vi "InAs TED Characterise - VoltageInput.vi"() -> ()   [LabVIEW 2024]
uses:
  <vilib>/Analysis/1siggen.llb/Ramp Pattern by Delta.vi
  <instrlib>/Keithley DMM6500 DAQ6500 Series/Public/Data/Read (Single Point).vi
  <vilib>/Analysis/NI_AALBase.lvlib
  <instrlib>/Keithley DMM6500 DAQ6500 Series/Keithley DMM6500 DAQ6500 Series.lvlib
panel:
  in  "DMM Visa":refnum<visa-resource-name>="DMM6500"
  in  "TEC Controller":refnum<visa-resource-name>="TED4015"
  in  "Average Filter Type":i32(ring) items=["Repeat", "Moving"]
  in  "Avg Count":u32=10
  out "InAs Detector Response":cluster{"Ramp Pattern":dbl[], dbl[]}(graph)
  in  "Tdelta":dbl=1.0 format="%#_13g"
  in  "TFinish":dbl
  in  "TStart":dbl=-65.0
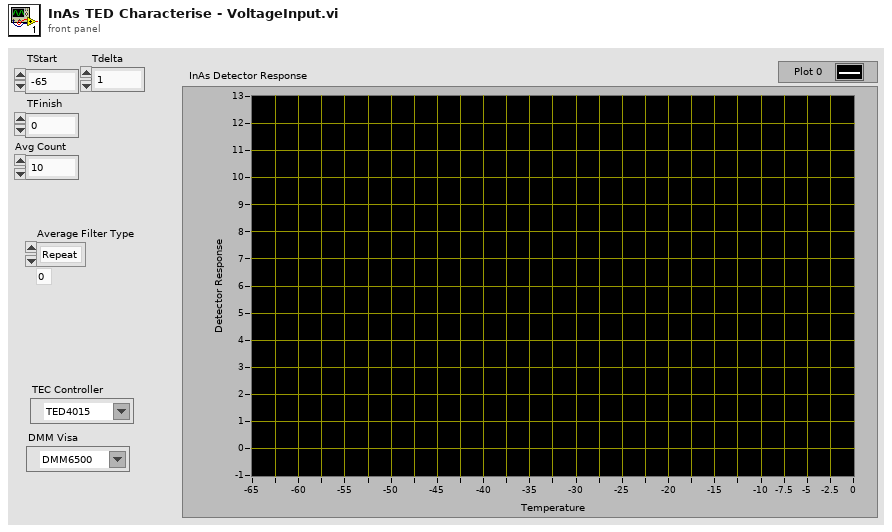
[diagram p1: front panel]
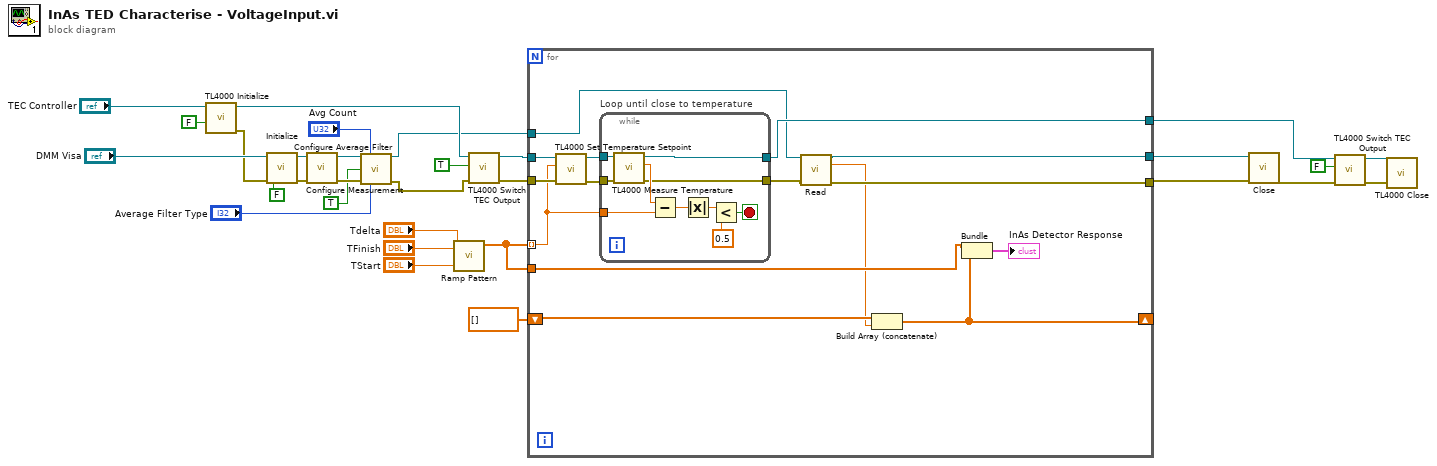
[diagram p0: block diagram]
diagram:
  n1 = call <instrlib>:"TL4000 Initialize.vi"("Reset Device (Reset Device)"=FALSE, "resource name"="TEC Controller") -> ("error out"=w27:errorcluster, "instrument handle out"=w30:refnum<visa-resource-name>)  [unwired: 8 in]
  n2 = call <instrlib>:"Initialize.vi"("error in (no error)"=w27, "ID Query (True)"=FALSE ("Reset (True)"), "VISA resource name"="DMM Visa") -> ("error out"=w9:errorcluster, "VISA resource name out"=w8:refnum<visa-resource-name>)  [unwired: 7 in]
  n3 = call <instrlib>:"Configure Measurement.vi"("error in (no error)"=w9, "VISA resource name"=w8) -> ("error out"=w5:errorcluster, "VISA resource name out"=w7:refnum<visa-resource-name>)  [unwired: 8 in]
  n4 = call <instrlib>:"Configure Average Filter.vi"("VISA resource name"=w7, "Count (10)"="Avg Count", "Enable Average Filter (F: Disable)"=TRUE, "error in (no error)"=w5, "Average Filter Type (0: Repeat)"="Average Filter Type") -> ("VISA resource name out"=w6:refnum<visa-resource-name>, "error out"=w4:errorcluster)  [unwired: 9 in]
  n5 = call-poly <vilib>:"Ramp Pattern.vi"("start"="TStart", "end"="TFinish", "delta"="Tdelta") -> ("Ramp Pattern"=w12:dbl[])  [unwired: 6 in, 2 out]
  n6 = call <instrlib>:"TL4000 Switch TEC Output.vi"("error in (no error)"=w4, "TEC Output (Off)"=TRUE, "instrument handle"=w30) -> ("error out"=w22:errorcluster, "instrument handle out"=w21:refnum<visa-resource-name>)  [unwired: 7 in]
  n7 = for {
    tunnel: w21 -> [w45]
    tunnel: w22 -> [w44]
    tunnel: w12 -> [w43] mode=indexing
    tunnel: w6 -> [w34]
    tunnel: [w32] -> w19
    tunnel: [w35] -> w20
    tunnel: [w40] -> w16
    shift-right: [w36] -> _
    shift-left: dbl[] [] -> [w39]
    tunnel: w12 -> [w37]
    n8 = call <instrlib>:"TL4000 Set Temperature Setpoint.vi"("error in (no error)"=w44, "Temperature Setpoint (25.0)"=w43, "instrument handle"=w45) -> ("error out"=w41:errorcluster, "instrument handle out"=w42:refnum<visa-resource-name>)  [unwired: 7 in]
    n9 = while "Loop until close to temperature" {
      tunnel: w41 -> [w49]
      tunnel: w42 -> [w50]
      tunnel: [w48] -> w40
      tunnel: [w46] -> w33
      tunnel: w43 -> [w55]
      stop <- w51 stop-if-true
      n10 = call <instrlib>:"TL4000 Measure Temperature.vi"("error in (no error)"=w49, "instrument handle"=w50) -> ("error out"=w46:errorcluster, "Temperature"=w47:dbl, "instrument handle out"=w48:refnum<visa-resource-name>)  [unwired: 7 in]
      n11 = Subtract(x=w47, y=w55) -> (x-y=w54:dbl)
      n12 = Absolute Value(x=w54) -> (abs(x)=w53:dbl)
      n13 = Less?(x=w53, y=0.5) -> (x < y?=w51:bool)
    }
    n14 = call-poly <instrlib>:"Read.vi"("VISA resource name"=w34, "error in (no error)"=w33) -> ("VISA resource name out"=w35:refnum<visa-resource-name>, "Measurement"=w31:dbl, "error out"=w32:errorcluster)  [unwired: 11 in]
    n15 = Build Array (concatenate)(w39, w31) -> (w36:dbl[])
    n16 = Bundle("Ramp Pattern"=w37, w36) -> (→"InAs Detector Response":cluster{"Ramp Pattern":dbl[], dbl[]})  [unwired: 1 in]
  }
  n17 = call <instrlib>:"Close.vi"("error in (no error)"=w19, "VISA resource name"=w20) -> ("error out"=w17:errorcluster)  [unwired: 9 in]
  n18 = call <instrlib>:"TL4000 Switch TEC Output.vi"("error in (no error)"=w17, "TEC Output (Off)"=FALSE, "instrument handle"=w16) -> ("error out"=w18:errorcluster, "instrument handle out"=w14:refnum<visa-resource-name>)  [unwired: 7 in]
  n19 = call <instrlib>:"TL4000 Close.vi"("error in (no error)"=w18, "instrument handle"=w14) -> ()  [unwired: 9 in, 1 out]
